vi "Set.vi"(6 "DC":i16, 7 "Channel":i16, 8 "error in (no error)":errorcluster, 9 "Range":i16, 10 "enabled":i16, 11 "Handle":i16) -> (0 "error out":errorcluster, 3 "Return Type":i16)   [LabVIEW 2023]
uses:
  ps2000.dll
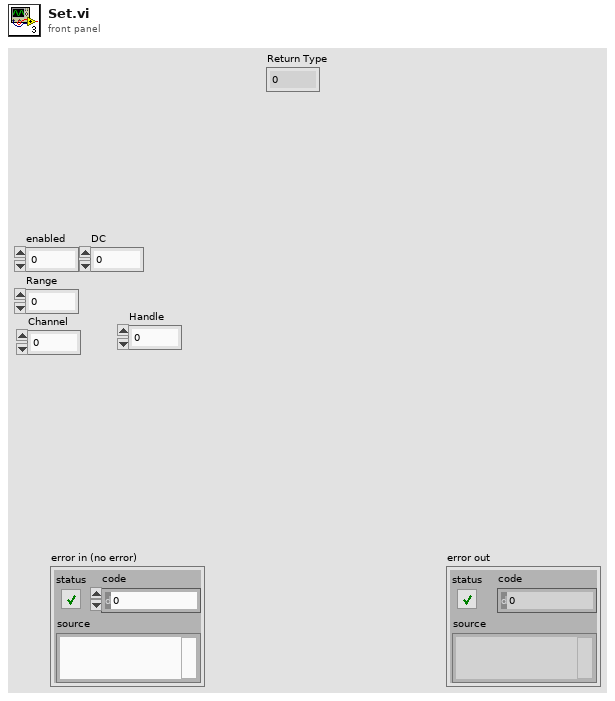
[diagram p1: front panel]
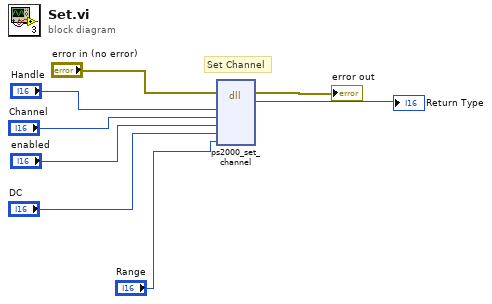
[diagram p0: block diagram]
diagram:
  # "Set Channel"
  n1 = dll-call lib="C:/Users/cesar/Desktop/Ps2000 libreria/PS2000.dll" fn="ps2000_set_channel"(error in="error in (no error)", "handle"="Handle", "channel"="Channel", "enabled"="enabled", "dc"="DC", "range"="Range") -> (error out=→"error out":errorcluster, "Return Type"=→"Return Type":i16)  [unwired: 7 in, 1 out]
